vi "UpdateCVT(Channel).vi"(8 "error in (no error)":errorcluster, 11 "TektronixDPO in":refnum<class "TektronixDPO.lvclass">) -> (0 "error out":errorcluster, 3 "TektronixDPO out":refnum<class "TektronixDPO.lvclass">)   [LabVIEW 2013, in "TektronixDPO.lvclass"]
doc: "Update the horizontal values in the CVT"
uses:
  TektronixDPO.lvclass
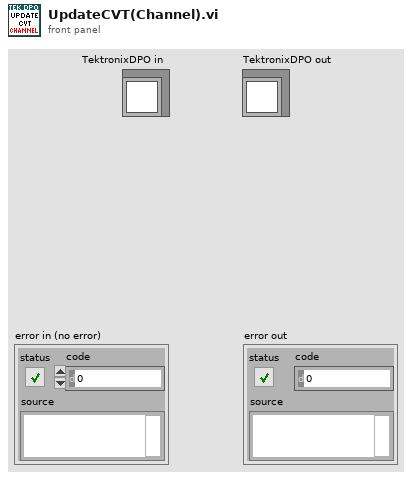
[diagram p1: front panel]
types:
  T1 = typedef "settings_TypDef.ctl" = cluster{"resourcename":string, "timeout":T2, "LocalSavingPath":path, "Save":T3, "Names":cluster{"Channel0":string, "Channel1":string, "Channel2":string, "Channel3":string, "Channel4":string}, "Calculations":T4, "NumChannels":T2, "NumMeasurements":T2, "NumPoints":T2, "waveformattributes":string, "Measurements":cluster{"Channel0":T2, "Channel1":T2, "Channel2":T2, "Channel3":T2}, "EnableMeasurements":T3, "Trigger":T10, "EnableReadWaveformInfo":T3, "probeattenuation":cluster{"Channel0":T2, "Channel1":T2, "Channel2":T2, "Channel3":T2}, "offset":cluster{"Channel0":T2, "Channel1":T2, "Channel2":T2, "Channel3":T2}, "Horizontal":T15, "verticalrange":cluster{"Channel0":T2, "Channel1":T2, "Channel2":T2, "Channel3":T2}, "Impedance":cluster{"Channel0":T17, "Channel1":T17, "Channel2":T17, "Channel3":T17}, "channelenabled":cluster{"Channel0":T3, "Channel1":T3, "Channel2":T3, "Channel3":T3}, "bandwidth":cluster{"Channel0":T18, "Channel1":T18, "Channel2":T18, "Channel3":T18}, "coupling":cluster{"Channel0":T19, "Channel1":T19, "Channel2":T19, "Channel3":T19}}
  T2 = typedef "BaseDriver.lvclass/numericVariable_TypeDef.ctl" = cluster{"Value":dbl, "Min":dbl, "Max":dbl, "StepSize":dbl, "Tolerance":dbl, "ValueActual":dbl}
  T3 = typedef "OnOffTypeDef.ctl" = enum16{"off", "on"}
  T4 = typedef "analysisTypDEf.ctl" = cluster{"Additional":T5, "Linked":T6, "Method":T8}
  T5 = typedef "additionalAnalysisCluster_TypDef.ctl" = cluster{"Analysis1":dbl, "Analysis2":dbl, "Analysis3":dbl, "Analysis4":dbl, "Analysis5":dbl, "Analysis6":dbl, "Analysis7":dbl, "Analysis8":dbl, "Analysis9":dbl, "Analysis10":dbl}
  T6 = typedef "LinkedChannelsCluster_TypDef.ctl" = cluster{"Analysis1":T7, "Analysis2":T7, "Analysis3":T7, "Analysis4":T7, "Analysis5":T7, "Analysis6":T7, "Analysis7":T7, "Analysis8":T7, "Analysis9":T7, "Analysis10":T7}
  T7 = typedef "channels_TypDef.ctl" = enum16{"Channel0", "Channel1", "Channel2", "Channel3", "Channel4", "Channel5", "Channel6", "Channel7", "n/a"}
  T8 = typedef "methodCluster_TypDEf.ctl" = cluster{"Analysis1":T9, "Analysis2":T9, "Analysis3":T9, "Analysis4":T9, "Analysis5":T9, "Analysis6":T9, "Analysis7":T9, "Analysis8":T9, "Analysis9":T9, "Analysis10":T9}
  T9 = typedef "method_TypDef.ctl" = enum16{"n/a", "max", "min", "energy", "trigger", "maxtime", "mintime"}
  T10 = typedef "TriggerCluster.ctl" = cluster{"Mode":T11, "Source":T12, "Coupling":T13, "Slope":T14, "Low Level":dbl}
  T11 = typedef "Choices.lvlib/Choice73.ctl" = enum16{"Immediate", "Analog Edge"}
  T12 = typedef "Choices.lvlib/Choice74.ctl" = enum16{"Channel 1", "Channel 2", "Channel 3", "Channel 4", "AC Line", "Aux", "Digital Channel 0", "Digital Channel 1", "Digital Channel 2", "Digital Channel 3", "Digital Channel 4", "Digital Channel 5", "Digital Channel 6", "Digital Channel 7", "Digital Channel 8", "Digital Channel 9", "Digital Channel 10", "Digital Channel 11", "Digital Channel 12", "Digital Channel 13", "Digital Channel 14", "Digital Channel 15", "RF"}
  T13 = typedef "Choices.lvlib/Choice75.ctl" = enum16{"DC", "HF Reject", "LF Reject", "Noise Reject", "AC"}
  T14 = typedef "Choices.lvlib/Choice76.ctl" = enum16{"Rising", "Falling"}
  T15 = typedef "Horizontal.ctl" = cluster{"time_window":dbl, "resolution":T16}
  T16 = typedef "Choice77.ctl" = enum16{"1E+3", "10E+3", "100E+3", "1E+6", "5E+6", "10E+6"}
  T17 = typedef "Choices.lvlib/Choice78.ctl" = enum16{"1M", "75", "50"}
  T18 = typedef "Choices.lvlib/Choice79.ctl" = enum16{"FULL", "250 MHz", "150 MHz", "20 MHz"}
  T19 = typedef "Choices.lvlib/Choice11.ctl" = enum16{"AC", "DC", "Ground"}
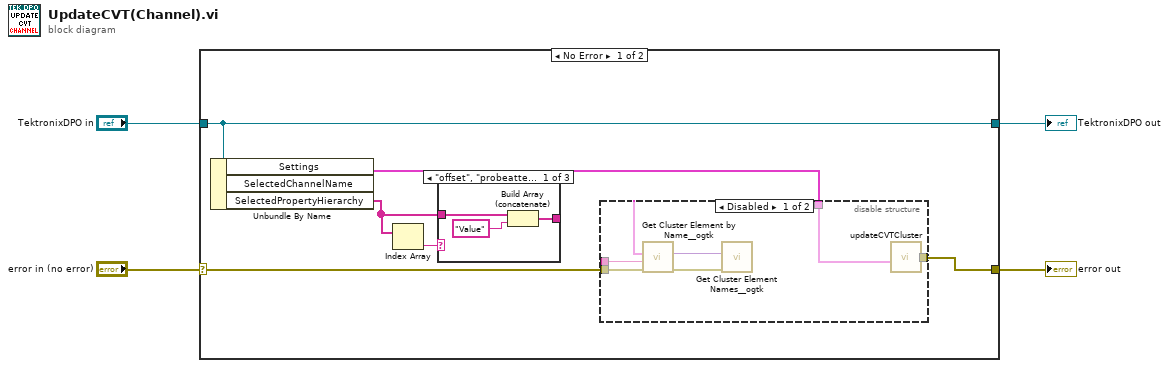
[diagram p0: block diagram]
diagram:
  n1 = case shown="No Error" "error in (no error)" {
    selector: "error in (no error)" -> [w8 w22]
    tunnel: [w10 w22] -> w4
    tunnel: "TektronixDPO in" -> [w9 w21]
    tunnel: [w9 w21] -> w1
    frame No Error {
      n2 = Unbundle By Name(w9) -> ("Settings"=w7:T1, "SelectedPropertyHierarchy"=w6:string[])  [unwired: 1 out]
      n3 = Index Array(array=w6) -> (element=w5:string)  [unwired: 1 in]
      n4 = case shown="\"offset\", \"probeattenuation\", \"verticalrange\"" w5 {
        tunnel: [w13 w14 _] -> _
        tunnel: w6 -> [w11 w14 _]
        frame "offset", "probeattenuation", "verticalrange" {
          n5 = Build Array (concatenate)(w11, "Value" ("element")) -> (w13:string[])
        }
        frame Default {
        }
        frame ? {
        }
      }
      n6 = disable-structure shown="Disabled" {
        disable-tunnel: [w20 _] -> w10
        disable-tunnel: _ -> [w19 _]
        disable-tunnel: w8 -> [w18 _]
        disable-tunnel: w7 -> [w17 _]
        frame Disabled {
          n7 = call <userlib>:"Get Cluster Element by Name__ogtk.vi"("error in (no error)"=w18, "Element Name"=w19, "Cluster"=w17) -> ("error out"=w16:errorcluster, "VElement"=w15:variant)  [unwired: 6 in, 1 out]
          n8 = call <userlib>:"Get Cluster Element Names__ogtk.vi"("error in (no error)"=w16, "Cluster"=w15) -> ()  [unwired: 8 in, 2 out]
          n9 = call "updateCVTCluster.vi"("variant (destination) out"=w17) -> ("error out"=w20:errorcluster)  [unwired: 3 in]
        }
        frame Enabled {
        }
      }
    }
    frame Error {
    }
  }
  "error out" <- w4
  "TektronixDPO out" <- w1
